vi "resize.vi"(1 "Array":u8[](array[numeric]) format="%x") -> (0 "MIMIC_CMD":string)   [LabVIEW 2014]
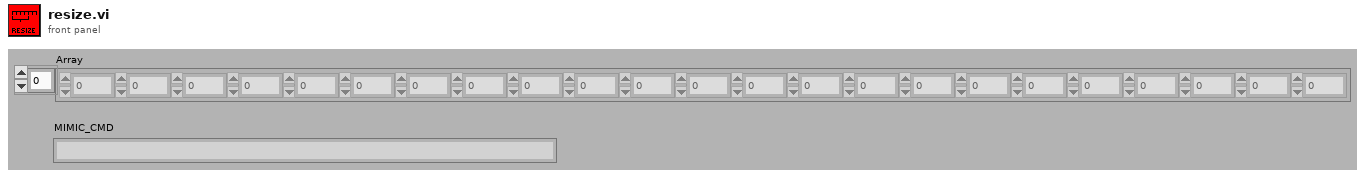
[diagram p1: front panel]
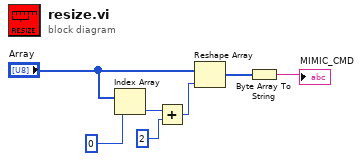
[diagram p0: block diagram]
diagram:
  n1 = Index Array(array="Array", index=0 ("Numeric")) -> (element=w4:u8)
  n2 = Add(x=w4, y=u8 2) -> (x+y=w5:u8)
  n3 = Reshape Array("Array", w5) -> (w2:u8[])
  n4 = Byte Array To String(unsigned byte array=w2) -> (string=→"MIMIC_CMD":string)
